vi "02_2.vi"() -> ()   [LabVIEW 2018]
panel:
  out "sum":i16
  in  "String":string="6-7 z: dqzzzjbzz\n13-16 j: jjjvjmjjkjjjjjjj\n5-6 m: mmbmmlvmbmmgmmf\n2-4 k: pkkl\n16-17 k: kkkkkkkkkkkkkkkqf\n10-16 s: mqpscpsszscsssrs\n3-9 n: wlxplcwkkqmdvnb\n16-17 x: mdxqxcxxxtxxxxxxxxv\n4-7 r: hrrrrxr\n3-7 d: ddndddcddddvddd\n7-15 p: rpjvppwfppsppptppqb\n1-2 n: ztznhmhldp\n6-18 x: stxxxxlptpxkxxxxxxx\n15-16 z: zzzzzzzzzzzrzzzz\n4-10 q: qqqpqqqqqqqbkdqrgqq\n14-20 m: mmrmmmmmmfmmmlmmzcmw\n1-2 t: qvxzmfgpxwgkt\n7-11 w: wwwwwwcwwwlwp\n12-13 g: gggsslggggggg\n9-11 v: vvvvgvnvhvvgvv\n1-11 z: tgksdczwmtzsfs\n13-15 t: hrshwjqvtlcqtrtttjhv\n4-13 h: hhhrxhhfhhmhhhhsdh\n2-3 s: shcsssss\n6-14 g: gggwgtgfpgqggwgg\n3-5 t: gsmtttttcbf\n8-9 b: gbbbbbbbbb\n8-9 f: ffqfffflf\n13-14 f: ffffffffffffnf\n13-14 v: vvvvvvvvvvvvhv\n2-8 m: mztxflwwrc\n1-2 d: ddddpfj\n2-7 f: fgffffgfffr\n3-5 t: htjxtstvtspttlxk\n15-16 f: ffffffffffffnfgtf\n3-11 p: pbgllspgppqhp\n1-10 t: mssrtttpzl\n3-4 q: qqcv\n4-5 s: dsscp\n3-6 n: nrjnnk\n2-5 z: zzzzz\n4-6 d: ddddwd\n4-8 f: zfqqdrfwcng\n2-6 s: ssnscs\n4-8 z: fzzzzvgbzwrzqzz\n14-18 z: thmkmmggvkfzbzfzvzt\n2-8 h: hhhhhhhh\n7-9 p: ppppppgpll\n1-2 x: cxkcrk\n1-2 h: lbrhhp\n6-9 k: kkkkkkkknk\n3-4 s: scjs\n2-3 s: fdshfsh\n5-15 s: vssspssssvkrlhk\n6-8 x: xtxxvxzhxxxxtxl\n6-15 c: ncccccccjccfclccv\n3-4 x: xxfcxlxxcxs\n3-8 x: xwxxxtkjxmtlxxxmx\n3-5 j: jjsjljzxjl\n3-12 n: nnlmnnnqgnmgs\n3-6 w: gwvswwww\n9-12 l: hlljlcklrcls\n2-4 x: cxfxqhx\n6-14 m: zrgnffnkcmntszgvnc\n1-6 g: gxqrgnzd\n4-9 z: zpzqzzgzzxxbzs\n10-13 l: jlvlllbxlvllt\n3-4 n: jxnx\n8-10 c: sccccczckc\n10-13 j: jkfgxjjjjjjjjjxzdh\n9-12 h: hhhhhhhhhhhhh\n6-14 p: hvpppxnpkpjbxpppppgp\n4-9 s: ssscsslsc\n3-7 c: cccccgcclqg\n19-20 l: ltfjvlllxhlnnlwlllfw\n7-8 n: nnnnnnnnjnn\n2-5 k: skntkhxkbwj\n3-6 z: pnzzzzz\n5-9 g: gpqtgggwxmghvgrqg\n3-6 k: khkkkkkk\n5-11 l: zlllljllnllllljhb\n6-9 l: lllllllll\n14-15 g: ggggggggggpxgkhg\n4-6 n: lgmntnxshxwpnq\n1-2 s: sxnst\n13-14 z: pwzstpdztzhwxk\n2-3 c: wmqrccn\n13-15 x: xxxxxxxxxxxvqxgxj\n6-8 b: pbbbbbbb\n8-19 f: prbsvkqfcdnrwhlnwfg\n7-8 x: sxlwxqxx\n7-8 p: xdtphpppqpppp\n1-5 p: cgplv\n4-11 k: kqnqkfkfxwk\n9-13 m: qhmnmsmmgmmmlm\n3-5 z: rzzrjxcqpl\n2-7 z: sjzcgsqqtfhnf\n4-7 c: vcpvkbbbd\n10-16 h: dspcrfnrthhvgcmh\n18-20 b: zbbbbbbbbbbbbbbbbbbm\n3-6 b: bbbbbbbbbbb\n2-4 k: kzcmhsv\n5-14 j: djcsjqjppfjwsjb\n16-20 g: gggggggggggggwgggglc\n3-4 g: gqggt\n4-6 l: llfjwr\n7-11 v: vvbmvlvvhbsvx\n1-18 p: nvwrgkkhschlrbbhkjqm\n11-16 z: zzzzzzzzxxfnzzzqzzz\n6-12 f: bxfsflvhfdrgftfsxvf\n5-10 r: trzwrbsrqr\n4-8 g: zfphgnjlgsbc\n16-17 v: vvvvvvvvvvkvvvvkv\n12-13 n: nnnnrvnknvnpdn\n5-9 x: xxjxxxxxw\n1-3 z: szxzz\n3-4 c: cccxc\n12-14 p: ppppppppwppppppppp\n19-20 p: pppppppppppppppppppt\n9-10 n: nnmnnnbnnnrmnn\n6-13 d: dbzdmdddvmdctwdbt\n5-9 j: jjjnjljjngkjjj\n5-8 q: qqqqhqqpp\n6-7 t: tssbttq\n13-14 r: rrrrrrrrrrrrrr\n2-6 w: wxwwmwww\n5-7 w: fwwlwwrw\n7-15 v: vvvvvvqvvvvlvvqvvsvv\n11-15 z: zzzzzzzzvzzsgzzgz\n8-10 f: ffffffffffffff\n9-12 p: pmrppppppppw\n3-5 f: kfwqw\n2-3 q: bkbqw\n9-10 m: mmmmmmmmvm\n5-17 f: wfqfnffffjwfvfffjbf\n9-10 m: mkmmpmmmbkmqmmm\n2-5 h: hhhthhk\n4-13 r: cklprhtqglcrhhrmqsc\n1-3 w: lwqw\n5-7 n: lmxnjknnlnnvbqw\n4-10 z: dlcpzqvjjq\n10-11 r: rrrrrfrrrrr\n2-7 h: hqtmfptxhk\n11-13 g: zmdlpghbsggbglxcjwc\n1-3 c: cnch\n4-7 k: kkknkkkk\n4-5 f: jwtffcfdff\n1-10 j: tjjfjjjzjbjjwr\n11-12 j: jjjjjjjwjjjjjjjjjj\n13-15 x: xxgxxxxxmxxxbxcx\n11-12 d: dcdddtdddddcdddj\n8-10 k: kpkkkkqkmkk\n5-6 h: mdmhjhhrhhdhhh\n13-17 g: ggggfgkngpggrgpgclg\n14-15 b: bbbbbpbbbbbjbsb\n1-7 x: wcqddxxhgmxxxvn\n8-10 l: lllhqlznjlllcll\n6-8 n: rnnnscnq\n14-16 m: fmmbmmmgmmmmmpmm\n5-6 c: vccccc\n7-10 h: vwgnhqhqhgpchhwhhhf\n2-6 n: ndwnnn\n1-2 v: vvvtr\n10-11 l: lllllltlllgt\n12-14 x: xxxvxxxxxxxxxx\n5-7 n: snnnnnnh\n3-5 l: rllmn\n9-12 s: jsssgsssftsvsss\n1-4 r: rfrrf\n6-8 r: rrrrrrrr\n3-9 g: rgpdqgsbfggflgbp\n1-15 t: tsbtrptnrtqtvtlgpt\n8-9 b: bblbbnbsbb\n11-14 g: ggggggggggwggcg\n4-5 c: scwgs\n8-10 d: ddkdxddddq\n2-4 m: gmmm\n3-8 k: wrkjkczkkgc\n3-4 h: sjhh\n2-13 t: tvttttttkttttttxctt\n5-8 p: plzpppppp\n6-7 q: qqqqpqxq\n14-18 r: rrrrrrrrrrrrrrrrrrr\n16-18 w: wwwwwwwwwwwwgwwmwd\n4-10 s: ssssjssshss\n7-8 f: fffhffgcf\n2-11 s: sdszssssqsntsz\n2-5 z: zzjjzw\n10-11 k: kkkkmkkkkzkk\n4-5 l: lllcdll\n1-4 q: qlrt\n7-8 c: cccccscc\n9-10 k: sxgqvkkkkkkkkzkk\n5-9 n: nnlkchnnnnwjn\n6-7 v: vdwvfdcbb\n3-5 q: bmqwtqkdbxzdm\n3-7 h: hhbhhhhhhh\n14-18 q: qqqqqrqqfxqqqqqqqq\n4-12 w: ndnwwcvfthhn\n4-5 b: bgbbn\n9-10 j: tjjjgjjjgjjgj\n3-4 s: svsm\n1-2 q: xfqqt\n7-8 p: fdpjsvps\n4-6 x: xpxxsxljlxxrxqjxp\n4-8 w: mbvdkwwwwwwhghlhj\n1-3 g: fngjxdc\n2-3 j: xtjjj\n4-9 j: lqphjhmgzjzjjvjjtv\n6-9 z: szzxzzqzzz\n5-11 c: cdccncccwfxc\n8-9 t: bttttttvtt\n5-11 l: rttpvrclsqfk\n3-18 b: hlwzvtqbbzbbbbvlvhb\n15-17 f: fffkffffffffffbffff\n2-6 l: lllqlt\n5-9 h: hhhhjchhhh\n3-9 x: xlgxxxxxr\n6-10 n: nnwxmxnpnf\n2-3 l: drlwrtltw\n1-2 b: gxbbrklvbsbbxbbb\n11-13 q: qqlvqqqqqqqqqqqqfp\n1-12 t: thdtvlgbstttmhgttbnt\n2-4 l: lllpvll\n3-16 t: lttpfnrgwdlkqtwgqrj\n7-8 d: ddddtdddd\n10-12 w: wwwbwwjwnwqwbwswwwg\n2-4 c: qqct\n1-4 j: jcjrjj\n4-5 l: lllbll\n11-16 g: ggkrgswgljjggmpzkg\n7-11 b: rbrbbczsbbbbbbfvck\n16-17 r: xfnpkmnzmlnrwrrrr\n8-9 x: xxxxxxxjz\n6-10 p: dpppdptpbpxpgbpppn\n4-5 s: scvcjsqssbs\n3-4 k: kktv\n8-10 f: fffffffffs\n3-4 g: gpbq\n10-11 x: xxxxxxzxhgdqxxvxxxxx\n7-8 g: nzgpgxgv\n4-6 n: nnnbzsnbh\n3-14 l: jdllllltlfjlld\n7-9 v: vvvvvfvvv\n5-7 s: ssbsssxjv\n6-11 l: xlllslrnlflnqhklllll\n14-18 x: xxxpxxxxxxxkxxxxxx\n10-12 x: xxvqxxxfxjxxxxxqp\n4-6 h: xfhhhhhhhj\n2-3 b: rbbbjmb\n7-10 d: dddddddddd\n15-19 g: ggggfgggjgggggggghg\n1-4 t: stth\n7-10 r: zskrphxkhgtmnsmzlr\n9-15 d: tkbdgngsddddrcd\n3-10 q: krqsqljqdfzqqq\n4-5 t: tztxtrgt\n11-14 z: jzzzzzzzzzzxzz\n18-20 p: pxpppbpppppppppppppv\n10-17 t: tttttjtttdtvvfqttxft\n8-15 j: vbjcjtdjzsjjjwjj\n4-7 d: ddddddd\n5-6 h: vmhlhj\n9-12 h: rhhrbhhhhhjh\n3-5 k: lkbkk\n6-11 d: dkfsjdmdddn\n7-11 d: dddddrsdddqw\n2-4 n: wnxngd\n12-16 c: cccccccbccccccctcc\n7-13 f: blfjmffffffwlf\n14-16 s: zsssssssrssssslrzfps\n5-6 t: tkkttt\n7-13 j: xjkjjrjmxjfpnvxqj\n8-14 c: cccccccckccccccsc\n11-14 k: kkknkkkkkhkfkxnkck\n4-5 d: ddddd\n4-5 w: wzmwwwww\n12-13 r: rnrrrsrvrrsrrrrrrr\n6-18 p: ppjppppppxppppppjppp\n1-5 m: gzhfjm\n2-5 s: scsrsssv\n7-10 t: tttthmztxbt\n3-8 c: crccmpwc\n9-11 f: ffffwmvffzfrzkfff\n9-10 q: vqvjtbtqkcnsbmfl\n4-10 l: lltlnfzxglwfxpgwntj\n2-3 c: pcccc\n5-11 s: jjgxwdfnsgjgxk\n3-8 d: vjqsdvjdhsx\n1-11 t: bjpthttlzttpbxtds\n7-8 s: sssssxsss\n2-6 b: qbzglpffcldtdb\n5-7 c: cccccvc\n5-6 f: fvffffz\n6-7 s: sspssdzhswsn\n1-6 l: wgdppqwnqp\n14-15 b: bbbbbbbbxbbbbbbb\n2-11 w: vqwtkmvbgrp\n5-7 w: wtwwwwwwwwww\n4-5 s: rsssss\n1-4 t: bwttt\n9-12 m: mmmmmfmmmwmn\n3-10 s: gmgjdslsnwsrv\n1-4 c: zsfcsrvsxczrgbtpwjkv\n11-12 f: fgffgtrfffksfff\n6-8 g: gggglbgg\n7-10 c: crcjtcccbh\n6-8 t: vjdktttttzcnthtwvtvb\n7-8 h: hchhthqhh\n4-10 k: hhkknpdlfk\n3-4 r: rrsjr\n7-11 g: ttrjggkdwbdnzmwzd\n5-8 b: nvqpcvfb\n6-9 b: bnbbbftbmbq\n1-4 m: smmmmmmmmmmmm\n16-17 p: pppppppppppphpppp\n10-13 f: ffwffffvmthvp\n9-12 n: nnvvcvmmfnnqnnsnnnn\n2-4 r: rrwq\n2-9 x: xzxxhxkxxtzdc\n6-7 t: ttrtltxt\n4-5 f: fffgxf\n3-6 v: vvvvvm\n5-11 m: mgxzmmgmlxxmm\n3-4 n: knnjcxn\n3-4 d: dndkgvkpbhdddcpt\n6-7 x: nxxxxtd\n11-12 k: kkkkkkkkkkmkk\n7-8 b: bkbbbbbzbbfmj\n2-5 d: drtdq\n8-9 q: qqqqqqqzj\n7-9 m: mkmmmmzmpfm\n3-5 b: bwcbv\n2-4 v: vvvvvvv\n5-6 h: hhhbbv\n12-15 g: gggggggdgtgqggngg\n8-9 l: llldllllll\n3-11 f: fdfpflzwfffct\n5-6 z: bhbzjgzz\n5-18 r: jtmnrhfrsptklgdksr\n7-9 d: llcrcqsfc\n16-17 l: kllllbllllllllllll\n9-15 g: ggvtgvgjggmgwslggm\n4-10 g: ggggggqgggqggp\n3-5 c: gchcc\n6-11 z: zzzzjzzzzpz\n3-16 h: hzhhhhhhhhhhhhhhh\n3-8 w: wwqwwwwdw\n3-4 g: wmklgdxxb\n2-5 p: ppbwqsg\n1-3 p: xpvpppppp\n13-16 x: pfqxdnxwxxzpxxvx\n3-8 m: qmlhjkzhm\n8-10 l: llllllfllll\n12-16 p: xtppfpfppppppdlk\n7-10 t: ttttttztmt\n11-13 p: pwlphpppcwnpv\n1-3 x: xxxx\n12-14 c: hcckccccccbvdz\n3-8 g: ggggggngg\n11-13 b: bbbgbcbbblxbbbbbb\n2-6 k: kkhhlhvtbd\n3-4 s: sstsss\n13-16 l: nljgklqlgfrlljtl\n9-14 l: llllllgllllhln\n3-15 b: bbtbbbbbbbbbbbpbbbb\n7-10 h: hhhhhghhhjh\n4-6 r: pnxrvrrnwrcrrw\n17-20 h: xbhcmhpvqzlhrbhhhbjn\n1-4 f: fffff\n2-4 c: vcclc\n11-14 f: fffgnffflffffff\n8-15 s: ssslsscwcssszsv\n7-10 r: drrbvtrphzqqrrsvncr\n12-13 l: vllllllllllbfl\n7-11 z: zwhzzhmqnbj\n6-11 v: vvkvvqhvvvjvwvvvvvvv\n13-14 h: shshhmhhhhhhfhvsr\n5-10 c: rwzcxwzvgcpn\n4-7 f: ckdfpmffpzlwjl\n5-7 x: xxxxkxgxxx\n18-19 x: xxxxxxxxxxxxxxxxxkxx\n4-6 r: nrcrdgrbrb\n9-12 f: ffffffwflffff\n5-10 z: zzzzzzzzzwzzzz\n4-5 d: dqmvqlhjxdkkdfn\n10-15 s: ssssssssssssssssd\n8-10 w: wpjvmwqwwz\n6-10 w: hxwxcwrqbb\n9-15 f: fffffffffffffbftb\n5-7 q: qqqqqqx\n3-5 t: wgbttttp\n12-13 k: kckkkkkkkkksztk\n12-15 w: wgwwwwwwbwwwwww\n2-3 s: tssstcph\n4-7 l: llllkll\n6-7 w: wkwkrxsj\n3-4 w: wkwwfm\n3-10 w: swtwckrrkwrvk\n5-6 w: wwwwwwlwjkknh\n1-3 d: dddd\n1-2 b: bcbj\n8-10 f: fffffffbvbf\n7-12 d: ddgvftsdrffbtd\n5-9 f: fffffffffffftf\n4-11 j: rbhjbkfjznjwqwz\n3-9 z: czzgzbhvz\n9-12 x: xxxpxxxwjxxvx\n3-9 k: zzkfjkcfk\n7-9 f: tffqcfgfvlffmd\n2-4 j: njzn\n9-10 h: hhhhjvhhhhh\n3-7 n: hndnbjdjx\n1-2 s: sshfsss\n7-14 g: kglngzbggggnvcgtgt\n11-13 h: hhhdnfhhhhqhhhhh\n5-6 w: twwwww\n5-8 j: fgxbqjjh\n7-8 f: fffffhvp\n3-9 j: pjjjjjpbj\n3-4 m: vmmsm\n12-13 x: xxxxxxgxqxxjnnx\n4-5 t: ttbbtt\n10-12 p: jjpppppcppppblpp\n9-10 b: wlbbbbjbbkbgnbbb\n6-8 t: tttstttzt\n6-9 n: fqxlnnnmn\n4-5 k: gwdzkk\n4-11 t: ttthktthtttbt\n2-4 r: rrpcnhrktrl\n7-9 j: hjbxdqbbmxmm\n3-7 b: bbbzqbbsbh\n15-17 s: sssdssspssssssgssss\n6-11 w: wwwwwpwwwwdww\n14-16 s: sssssssssssssgsrs\n2-8 z: kzbzbzthzgzzwcw\n11-13 q: qqqqqqqqqqjwq\n3-4 v: dspkvr\n1-5 n: nnnnnnmn\n4-5 b: blbbsbb\n5-7 r: rrfrkcr\n5-6 c: zpcrlp\n15-16 b: bbbbbbbbbbrbbbbg\n5-6 j: jjjjrcjj\n9-12 z: mzgnzzdjzzzzzdzlzzzz\n5-7 z: gztczpzbzdzlzcjzj\n6-8 w: hwhwfmswrrcpxlsqlkkd\n6-11 p: pppsppmpnpp\n1-2 w: vdwl\n8-13 m: mmkgmmlmnmmvm\n2-3 q: qqqh\n2-5 x: xxxxrmxxxxxjxnxxcnd\n7-8 p: fwpppptp\n2-10 l: lllbhlltclln\n10-11 v: vvvvvvvvtrgvv\n13-16 m: mmmmmmmmmmmmnmmmm\n3-4 n: qtfn\n7-8 g: gggwgggw\n10-12 n: xnnnhcqhnnnpnphnnnnx\n3-4 q: qrqq\n4-8 c: cswcccclzx\n2-8 h: hphhhhhd\n1-16 r: qrfrfrtgrrrxrrzhbg\n11-12 q: qqqqqqqqqqqqqqqq\n10-11 v: vvvvvvvvvdf\n6-8 n: lnnrnnwnnldmwn\n1-5 j: jjdkfgkjvjjjjj\n14-15 j: jjklzggckqksgvk\n10-11 g: ggggggggnzng\n15-17 n: ntnnllvnmbzwnnhzw\n13-16 g: gggggggggggqdgghc\n12-16 g: sgggggggglggnggggggg\n3-4 x: xnplx\n5-9 m: mjldmlmmmgbmjsbkm\n18-19 h: hhhhhhhhpzhhhhhhhhh\n9-10 f: ffbfffdfjf\n8-13 s: gssghjssgxsgssgsnj\n2-5 m: mmmmbhdzkmmh\n8-18 l: hqnqzznqkmskljggbl\n2-3 m: nfjm\n1-7 z: dnztzkpfwv\n2-9 s: ssvsdvjwdsw\n15-19 f: fffffffffffffcsffcn\n13-20 c: ccccccccccgccccwcccc\n3-15 b: bwmzdgbbjvbbbrt\n10-13 d: ddddddgcddmdhdd\n4-7 h: hlhhhphz\n2-3 c: cccbgfbzdql\n13-14 w: wwwcwwgwwwwwcqwzw\n2-4 m: hmmlmmmmmm\n3-16 x: jzxcfkxzxcvfxwxfxx\n3-8 f: kfpffvfwfkf\n8-10 q: pqqmlqqcqqqqf\n3-6 r: qrfcrrwqcrrbttrb\n3-10 s: kdstdvqqdcb\n11-12 f: lcxfllffffffflffff\n4-8 m: mmmmmmmzmmmmm\n6-8 w: wwwwwswwdw\n10-15 b: bhfbbjclbbhwthxltsjn\n1-5 v: dvxvw\n13-16 s: ssssssssssssksswss\n6-7 d: dlfldrt\n4-10 x: xxxxpxqxgxgrh\n4-8 x: xxxxxxxxxx\n4-5 r: vrxrrrrrkxrp\n3-14 h: hfmpnxlklhhhjhzh\n11-15 d: cgddqnxgddddzrdd\n7-12 v: csmfvjvlvzjv\n4-5 g: ggngh\n14-17 z: vzzzzzzzzzzznvzzzb\n15-20 q: qqqqqqqqqqqqqqqqqqqn\n1-3 x: xbxqnzhjzhbxbbnsnt\n11-13 d: sfdtlhdddjkshd\n11-13 c: vbtcncclfzmcc\n1-7 t: ptttttqtt\n3-4 x: xxsxx\n1-2 h: hjhh\n10-13 f: vlcfqpwgqfthf\n14-19 w: wtswwwwwcwwpwswwwww\n7-10 h: fhxhhhhlbw\n4-14 k: khfkkckvkdxkfkvp\n4-6 k: kknkkkbk\n3-14 m: mhvdmpnmwvkcmgbbv\n17-18 h: hhhhhhhhhhhhhhhhrs\n16-18 c: cclccccccccccccxcmcc\n9-12 j: vjjjljjjqjjjjq\n2-3 d: dlrbddmj\n10-15 l: lllmlllhllllllll\n1-2 n: nbnd\n8-11 b: wvbbbbdbbbbbpxbbb\n4-5 c: mccccfcc\n2-12 d: kbdsddgddpwddzx\n9-10 t: ttttjttttbtt\n6-7 j: jjthjvwj\n2-7 l: lglqllxlh\n2-4 t: tnqjb\n1-8 c: nqrbcgbchxwkjrxv\n13-18 c: ccxmccccccccdcgccn\n9-10 s: shsssgsgssksl\n4-9 n: nnnxnnzngrpxn\n10-14 x: jprjxdlnrfwnqx\n1-5 b: bsshbls\n1-4 n: nttnmbblbntbssqn\n8-9 x: xxxxxxxxxxx\n2-4 c: nnccmp\n1-14 t: stttztttttlttq\n9-16 b: rfbmptrnbhwbrgbbqb\n1-4 f: rzzfjkmnwlbnrqmfns\n1-3 x: mxxdlxnklrktlgzd\n3-13 v: zlnktcwvmkqsvjvnwzv\n1-3 r: rrrrr\n5-7 d: qdddcddldd\n2-5 t: tnttktt\n8-15 n: ngnnnnngnnnnnnn\n1-2 v: vfvn\n3-17 f: ffffjfffffffffffgff\n5-12 x: nxxxxxtxxrxxx\n2-14 g: nfgvdgnhggrgtkv\n11-12 k: kkkkktkskkkkksm\n15-16 c: rccccccccccccccccc\n10-12 l: cllwldllplsl\n15-19 b: qbjbpbbbbbbwbbgbbcq\n13-16 f: dqcfgwfffffffffb\n3-4 q: qtzj\n13-15 z: zzzzzzzzzzzvzzzz\n13-18 q: qqqqqqqqpqqqqhqjvqsq\n7-12 r: dtflckrndscrqrcclxb\n4-9 s: zqsssshqscs\n2-5 s: ssrhsfsszsc\n7-8 k: kkkhkkwzktkkk\n17-18 x: xxxxxxrxxxxxqwhklp\n16-17 k: kkkkkkkkkkkkkkkkrkk\n9-11 s: szqfssvgfvm\n11-17 m: mmmmmmmtmmmmmmhmpmmk\n6-7 l: kgllhjdllwqvllnlcn\n1-2 g: gghgfgv\n4-5 f: qfrrrlfrtfzgfct\n6-7 z: zvzzzzj\n7-12 m: lmhzrxztktzpkvw\n3-4 p: ppxpp\n4-5 c: wvxch\n9-12 x: xcxxxxzxcxpxx\n10-11 t: tttttgttttl\n2-3 w: tcwdwb\n1-8 m: mnsmmmmgmm\n1-5 z: zzzzz\n2-13 j: jvjjjljjjhjjjrjlj\n4-5 s: kcmxszckjcsswjbsxn\n6-7 j: dhjccbb\n15-19 x: xxxvxnxxxxxxxxnxxxx\n15-18 f: ffffrffsfffffjffsff\n8-20 m: xmcwmmmhsmmmmmbmmmmm\n8-14 m: mmmmmmkmmmmmmm\n2-6 r: bnrrrv\n8-12 k: kkkkkkkjkkkpkkkk\n1-4 f: flqfgnffzjrfz\n2-6 p: pcvgxpnl\n9-12 n: nnnnnnnnkgntnn\n13-15 h: hhhhvhhhhhhthhhhwphh\n6-7 h: hhhhhhkh\n8-9 h: vhhhhhhhhh\n1-5 m: mbmmmszqwmxdhd\n5-6 v: vvmbwvv\n4-6 g: vggttg\n8-15 t: dzkznmcvqmbbtxs\n13-15 j: jjjjjjjjjjjjjjjj\n5-11 r: ptwmxlrttvxk\n10-12 s: ksszsbqxsjsssnjst\n3-4 k: jwkr\n3-6 m: mmtkmmm\n2-4 l: lhlll\n7-12 p: pppppprppppzpp\n1-2 n: bznpdd\n11-13 t: ttttttttztdct\n6-12 c: cccccdccccccc\n2-7 n: nznnknrnnn\n14-15 h: zqxhdhhxhhhhhzpr\n6-7 x: xxxxxjx\n5-7 s: gsfcshsbxnc\n12-13 j: jjjjjjjrjjjjjjjjj\n4-5 v: vvvvc\n4-10 r: rrsrzrhrrgrmvrs\n8-12 c: cccwcccccccmc\n4-5 v: vvvvv\n13-19 j: lfnkrsjjjjjrjjzgcmj\n3-4 k: kkskkk\n11-14 s: sssssssssssssssssss\n8-9 k: kkbkknkkk\n4-6 z: zzzqzqxzz\n2-4 f: rgtz\n4-13 k: kkkkjkkkkkkxk\n1-6 q: jqqqqpqqqqqqqqqqqq\n7-9 b: bbbbbrlbj\n4-5 j: mgjjtjfs\n15-16 p: ppppphppppppppnpp\n2-3 b: btbt\n11-12 v: vvvvvvvvvvzk\n1-4 b: qbbbh\n6-7 b: bsbbbbnwb\n3-10 j: gkjrhtjjfjjjrjjjjrw\n4-5 g: gdgqtpgg\n15-17 g: gggggggggrgggggggg\n1-3 j: hjdjpj\n5-6 k: jjslkhnwkfqjprk\n7-10 s: ssscssssnsx\n1-9 n: nnnnnnnnnn\n1-14 t: ptttttttttttttt\n11-13 q: qqqtqqcfvqsxzqqqqqq\n14-15 r: rrprsrrrqmjbrrv\n4-5 h: hhhhdhh\n5-8 l: lllllllll\n18-19 f: fwfffffffffffffffff\n9-11 j: zjnjjvjjfbj\n3-7 p: sjpsmsc\n10-11 s: sscsssssrrls\n3-9 q: qqqqqqqql\n6-20 s: sqscdsmdgvddfsvprgcs\n18-19 q: qqqqqqqqqqqqqqqqqqq\n4-5 g: mgjggnjfgl\n3-5 p: ppcpzp\n14-16 t: fjxbttlttfprttlt\n4-7 v: pzmvzvlzxcccvmvvwfdb\n1-8 r: rkrrtkrrgrrq\n1-10 h: qhhhhhhhhdf\n1-4 p: rpppp\n4-6 s: skshzg\n16-17 h: hhhbhhhhhhhhhhhch\n2-10 m: mrmpvlsxvtlkwpnl\n7-10 b: bbbbbbbrdb\n15-18 j: mjjjkgmjjbjjjjcjjmjj\n3-6 m: mgmmdmmmj\n5-11 n: ktnnwnnntznqnnnpnnn\n9-12 w: wwwwglwwzwwtww\n8-9 t: ltttvttvv\n4-8 c: xdfklzfhgjgcktssk\n7-11 x: xxgxxxxzxmxxxxqcc\n13-17 v: vvvvvvzvvvnvvhvbtv\n13-16 c: ccccccccgccccccw\n3-13 m: mmkpmqjkdknmmrmfcm\n7-11 g: gpgsvmgvdkg\n9-14 g: gvgglglghgjpwjzgsfh\n2-3 v: vvcv\n3-8 w: zwqjwwwwwm\n7-9 k: kkkkkkzkb\n3-4 v: gvvk\n14-15 r: rrrkfhmpgbhtqrh\n4-5 n: nnnmwnn\n7-9 l: llltdlvlx\n6-7 f: ffffffl\n7-8 n: nmnnnwfg\n17-18 x: xxxnxxbwxxbxxxggvxx\n1-3 z: cbzntpzvgpszsdq\n3-4 j: jjjj\n3-5 z: zznzgz\n4-5 j: jjjcg\n7-8 j: mjjkjjxhj\n1-2 t: vrlmttt\n3-4 h: hhhhhrhhhphhh\n14-20 q: qqlsqqqmqqqqqqqsqjjg\n9-10 r: rxrrrrcxrbrrnsc\n8-15 x: ghlzxrvjvjxrndvknxxt\n1-3 b: bbbb\n4-6 t: fnqthtnfjprghdmt\n6-7 m: mmmmmcgmm\n6-8 q: bqqvqvqd\n7-16 v: vvvvvvvvvvvvvvvvvv\n3-4 p: ppjlppppppppxlztpp\n12-14 g: ggggnrggvgggmgg\n1-10 k: kxkktkkkpkkgt\n4-5 z: zzwrw\n14-20 p: pppppppppppppspppppp\n6-11 t: hkbbtbmrdlkjlthgkc\n6-13 f: fpcfzfcpfjqhqwffffd\n2-3 h: hhhjhh\n3-4 z: ztcbz\n6-9 q: kqlqgtqwvxcgqwqr\n9-14 k: kkkkskkknkkckjk\n14-16 n: nnnnnnnnrnnncprcnn\n1-9 m: pwwmgmxmnmm\n1-5 f: fnmpfc\n3-5 s: jmsls\n5-7 b: bbbbbbbbbbbj\n4-12 m: gjzqmjktbrbk\n4-5 k: krkkkk\n3-10 q: qqcnrqqqbnqq\n1-2 s: gvsk\n5-6 n: nsjnnn\n1-5 w: wwkwztqc\n4-17 z: zbbnqfqmrjbszpwxz\n2-9 z: djpdvrdbx\n2-4 w: lwxw\n1-10 g: gsgpgggrgggtgwsgg\n3-6 q: qqtqqq\n3-7 x: xdxxxxx\n1-2 t: ttft\n4-6 x: lxjxsxpvxxxkjqlsxndf\n1-8 r: rbzrrrrrrsrrrrrv\n1-6 g: gggggggggggggg\n2-3 q: smbbmntqr\n8-9 d: bzmplgdfq\n5-10 w: wwwdwzjwwwww\n2-11 z: jzgphzdjwxw\n9-12 d: dtvdddjdlddddd\n5-16 s: hswkqwssjshpsxkgmsw\n3-13 c: cwbcccccccccgc\n2-13 b: bhswhcxchtknt\n1-3 h: hhhtmclgrtxdvqfpk\n12-13 w: bswxxxmxwjtwp\n4-6 c: xtcccc\n6-16 k: msskfkgdkpcnqtzkpqh\n6-7 t: tpttftt\n5-7 h: hhhhhhh\n3-8 t: tbrshhlt\n8-10 j: jjjjjjjhjjjjjjjjj\n11-13 g: vgwggggggkshjggnqggs\n6-10 q: jqqgzqpwqqfqqqd\n5-12 d: ndwgszjhhdwv\n4-5 t: tttmkttt\n2-3 p: ppwp\n7-8 t: ttttttzb\n13-14 m: mmmmmmmmmmmmpxmm\n5-9 v: cqvbqvzzvtcdnvvvbz\n10-12 q: xbfpjqpzlqcq\n8-10 l: lhlkllclll\n4-15 t: wjtqftxkskpvttxmb\n1-5 s: lzscqfrpfss\n7-9 x: xmvxfxxjx\n6-7 w: wwwmwwwwww\n13-16 d: kbddtmrdqgqqddhd\n1-17 q: vqqqqgqqqqqqqqqqqqq\n3-5 f: nkftsfvzc\n4-7 h: hhhhhjrd\n5-11 z: zzzzzzzzzzlz\n4-7 k: kkkkdkkk\n17-19 n: nnnnnnnnnnnnnnnnwncn\n8-16 r: hpvsmthdvmxrbqvr\n2-10 b: bbrxblvbbdvcbdbbbqsb\n8-11 r: rrrrrrrzrrv\n1-2 r: vtrr\n2-3 m: mmcmmmm\n3-10 c: xccccscccc\n10-11 w: wwwwwwwwwwzw\n3-18 f: fspffffffjpfffffff\n4-16 q: kqqqqqqqqqqqqqqkqq\n10-11 l: llllxlllldv\n13-19 t: ttttttttttttttttttt\n9-12 d: drddddddmddd\n5-6 n: kngrnn\n5-9 x: sbxxxtkvpjfxxxv\n8-11 d: dkwddrdrdddd\n8-11 d: ddsddddhdbd\n4-5 l: pxlll\n12-15 m: sjlnmmhndcmmzrmm\n7-9 t: ttttttdtctt\n3-5 n: snfxc\n4-5 l: lmpll\n5-10 z: zzlztzfttxzfprz\n13-14 d: ddwjdqvjdddvdj\n14-18 r: rrrrrrrrrrrrrgrrrhrr\n4-6 g: ggggqc\n9-16 m: mmrmmmmmmmmmrmmm\n1-8 f: fffffpfkffff\n7-8 b: bbbbbbdtbbb\n5-8 k: hkkbkkkkkkwk\n9-12 d: dhdddqdhddkddddddd\n10-12 r: rrcrrxrrrgrr\n6-7 r: rrrrrrrrr\n12-18 c: cccccccccccccccccc\n1-3 x: glnwxx\n4-12 s: splscqfbvbvswgrvvhg\n7-14 n: nnnnnnpnnnnnnb\n4-8 x: xlqxbrkx\n11-13 t: ttttttttttktv\n1-7 w: wwgwwww\n8-13 p: lpzxtppplplff\n6-7 q: qqwpkqqqqz\n4-5 j: zdkmjrpjlzbjprv\n4-6 x: xhtxxxg\n2-14 j: jjjjjjjjxvjjtjjjwj\n8-9 d: gddddndcgtdn\n4-7 g: gglgpgr\n7-10 d: drddddsddd\n1-3 n: nbnnb\n3-4 k: dggss\n6-10 t: cwcwtnttmt\n3-4 x: xxxx\n8-12 t: jttmtbttqtztttzmtc\n8-10 t: tttgtttztttg\n3-4 h: hhhhc\n10-18 t: tttttttttmtttttttbtt\n3-5 n: nnnnnnz\n4-12 w: wwwwqwwwjwwxwlwqww\n2-4 x: xqdpr\n9-16 k: kkkkfzbkkkknjknkkr\n2-7 t: tttttwt\n2-4 p: npjp\n5-12 c: cccccccccchxcc\n9-14 x: xvbxpxxshxnmxzxxxwn\n10-11 t: ttqtvttjtcttmtttt\n9-15 c: cccbcxcswnrzchfcqwjc\n3-4 s: vpczjdzgfsqnpsscf\n7-11 b: bbbbbbtbbbb\n4-15 q: qqqzqqqqqqqqqqqqqqqq\n2-4 s: fsvsmlsfbgz\n1-8 w: wbwwwwwtww\n8-9 w: phbxcfdwwhrbhkgrzdx\n6-9 x: xxdpxhsxxxkx\n5-9 b: bbbbfbbbsb\n12-18 m: mmmhmbmmmfmrmmmmmmmm\n12-14 l: lllllllllllllll\n8-11 z: zzzzzzzzzzzzzzzz\n2-3 d: dlld\n6-7 b: kghbbbbbg\n18-19 c: cccccccccccccrcccccc\n6-8 m: mwnpmmjmfmmmfmhjf\n1-5 j: gjjjxl\n3-4 p: pzpppppp\n12-17 z: zkzzzpzzzzzndzzzzzz\n13-18 k: knvkkkzvkkkkkkwkkmkc\n3-4 h: hfgrm\n2-6 z: xzzzvzkzzzzvprtgz\n12-19 b: bbbbbbbbbbbpbbbbbbdb\n3-11 v: xvrvmvvvfgzvjv\n7-10 r: frrrcrrrrrrzr\n1-17 v: vhpxjwbpkcctdpsvfkxs\n3-8 d: hbdzlkdk\n5-6 f: flffzf\n2-4 s: ssnsssh\n4-5 m: qmffj\n6-11 z: zzzqztznfzzkc\n3-4 m: tjkm\n2-4 n: nnwn\n4-5 s: npxck\n16-17 n: nnnnnnnnnnnnnnnpk\n10-12 s: ssssssssssss\n2-4 g: twghtgs\n9-11 w: wwwwwwwwdww\n15-18 h: gfvmkzsrczchxwfvdr\n9-10 p: ppppppprtp\n4-5 p: pppgf\n2-11 c: qccccrsbjbsxbnjx\n8-9 l: lllllllvl\n10-15 s: sksssssssssscssss\n4-8 k: kfkklhgk\n5-9 t: ttgndtthqcfj\n2-3 t: spntttnqdttjt\n12-16 t: tttttttttttttttttt\n19-20 j: jnjdjbzjpjjnjjrjjjdj\n2-6 c: rrbhhggnnzcjvp\n7-13 r: rrlrrdrrrrrrr\n2-8 f: dfsvpmqfbqc\n10-12 p: bpprppnbprpppp\n4-6 z: lzszznzzxxzzm\n2-5 v: vmvvv\n9-17 v: vvvvvxvvvvvvfvvvf\n6-10 t: tcflkttctht\n10-16 d: qbxwwbqdxxlqtndktlx\n1-8 g: ggtgggcgggggr\n1-2 t: tttqqt\n9-10 k: knkkcnkdkkzkkkq\n12-18 r: rrrrrrrmrrrrprrrrkrr\n2-5 x: xxxcxxxxxdsjx\n6-7 z: cvzzzzz\n5-8 b: qjpzdbdx\n19-20 n: nnngnnnhnnnnnnpnnnwp\n3-19 g: vgggpxgnfkhvdrgggsng\n3-5 b: bvbbqh\n3-8 h: hhghhhhhhhhhhhhh\n2-4 x: xxtxfcppsvxrdtnjgs\n6-8 x: xxxxxxxx\n1-4 k: kfzkbkkkt\n17-20 h: hhhhhhhhhhhmhhhhphlh\n5-7 b: tfbvbrc\n2-4 f: ffcgfzfrmfsft\n18-19 t: ttfttqklqvgtkltnlgn\n1-4 c: tctc\n8-18 g: gkndqqgdgqrgkzgggg\n11-12 b: bbbbbbbbbbbpb\n5-9 t: qgtntdbdw\n1-5 n: nqnnnnkns\n1-3 c: bcccqccccw\n8-13 l: lllllmpkllllwhl\n7-10 c: czcsbcnccqwcsgxpcw\n3-5 h: bhhqjjpnh\n9-10 p: pppppppppw\n4-5 x: xxxxf\n1-5 h: mhhhhhh\n1-17 c: hcccckccpccccfccc\n8-9 p: pdgpplpppp\n1-7 r: rrfrrrmrrr\n3-18 x: xxxxxtxxxxxxxmxxmlx\n1-4 t: fttt\n9-14 x: fxxcxmzqgzzjktddmcf\n3-4 t: tttt\n3-5 l: lljmk\n1-3 g: dswcw\n7-8 l: ltlxlnllll\n2-4 q: lqvqpjcqfk\n2-7 r: prrrjbrrlmrbb\n4-7 b: bbbbbbbb\n5-6 k: krhkkkkkkk\n2-6 x: xxxxxxx\n6-12 t: xmttzbtspxgd\n1-8 x: xxxkxhxxxxx\n7-12 r: rrrrrrzrrrrq\n17-18 k: kkkkkkkkkkkkkkkkvsk\n12-15 j: zjbctccpfljrzbd\n9-10 z: zzzzzzzzzmzz\n1-4 l: crmn\n6-15 k: nkknzkkrgkcnkds\n3-9 z: zzzzzzzzzz\n2-10 v: vvvtpkxkvvvvzvvvvvvv\n1-2 h: hhhsn\n2-4 p: qgpgp\n2-4 p: dvqjxdwnvrkpg\n15-16 p: nkprmxpxpxhvpcmw\n16-18 b: qbbbbbfbbbbbbbbnbd\n4-5 t: thtxt\n2-7 g: rpvlhbdw\n6-7 k: kkpxdkg\n7-9 n: nnnnnnqnz\n17-18 h: xnmkfwtzflhkpsjthhbl\n3-5 k: kkdkm\n14-15 h: hhhhhhhhhhphhhchzzt\n6-13 j: jjjjjjhjjjjjjjk\n2-4 x: xxxwxx\n1-2 s: ssws\n4-5 m: fmztq\n5-6 p: ppppld\n3-7 w: wwwwwwww\n5-7 d: vgfddxdzvkndndzm\n1-10 n: nnnnnnnnnnnnnn\n1-9 q: gwmrrblpmqlqpqgqqmqj\n2-12 s: mqspzltmqsngwmlmk\n3-9 w: twhfxnkmw\n12-13 c: cczcccccccccl\n2-4 d: dpdtdqlssxddddddhd\n1-2 w: jqvw\n6-14 n: nnnnnjnnnnnnnnn\n6-7 b: bbbbbbbb\n14-16 z: zbvzzzzzzzzzzzzzzzzx\n7-12 f: fffnfffdfqfffg\n1-2 t: ftttt\n5-18 d: dtcdddjvdxddsdtdkk\n15-18 s: szsssssdsssdhstssp\n6-9 m: lmmmmmmmgljm\n2-6 n: nvsnjg\n5-6 l: lllhvx\n16-18 r: rrrrrrrrrrrrrrrhrr\n1-2 b: qbkbb\n10-18 x: gfjmjtbxxlxmxzxxql\n2-5 c: cdbjm\n3-4 k: rsvvwknnkjvwnkkf\n1-3 b: mbbbbb\n3-4 c: ccccc\n3-4 x: zxtkxn\n2-10 d: dbdddqtdxvjq\n8-11 k: kzkkpkkbkzq\n4-7 h: hhxhzmwhhhh\n11-16 r: rrrrrrrrrrrrrrrlr"
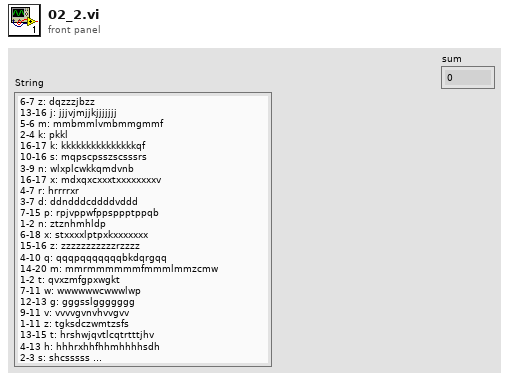
[diagram p1: front panel]
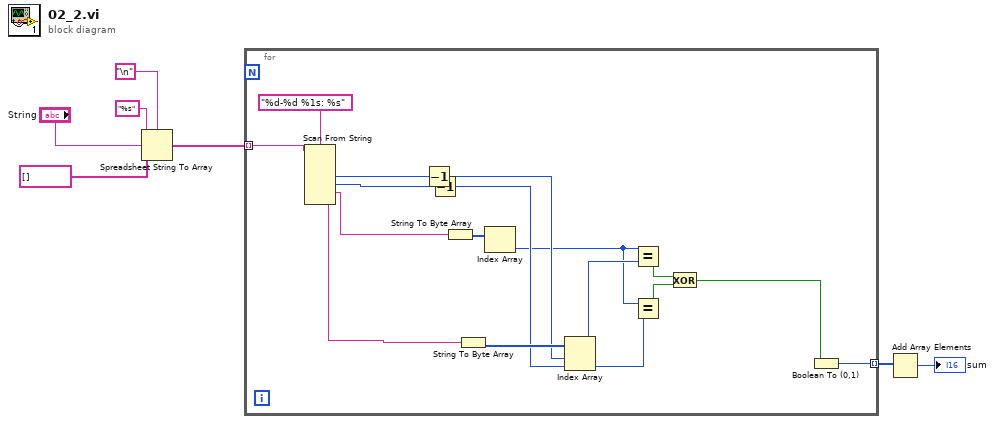
[diagram p0: block diagram]
diagram:
  n1 = Spreadsheet String To Array(delimiter (Tab)="\n", format string="%s", spreadsheet string="String", array type (2D Dbl)=string[] []) -> (array=w3:string[])
  n2 = for {
    tunnel: w3 -> [w24] mode=indexing
    tunnel: [w19] -> w2 mode=indexing
    n3 = Scan From String(format string="%d-%d %1s: %s", input string=w24) -> (output 1=w17:i32, output 2=w16:i32, output 3=w21:string, output 4=w22:string)  [unwired: 6 in, 3 out]
    n4 = Decrement(x=w17) -> (x-1=w15:i32)
    n5 = Decrement(x=w16) -> (x-1=w14:i32)
    n6 = String To Byte Array(string=w21) -> (unsigned byte array=w20:u8[])
    n7 = String To Byte Array(string=w22) -> (unsigned byte array=w18:u8[])
    n8 = Index Array(array=w20) -> (element=w12:u8)  [unwired: 1 in]
    n9 = Index Array(array=w18, index #1=w15, index #2=w14) -> (element #1=w13:u8, element #2=w11:u8)
    n10 = Equal?(x=w12, y=w13) -> (x = y?=w10:bool)
    n11 = Equal?(x=w12, y=w11) -> (x = y?=w9:bool)
    n12 = Exclusive Or(1:w9, 2:w10) -> (0:w8:bool)
    n13 = Boolean To (0,1)(Boolean=w8) -> (0, 1=w19:i16)
  }
  n14 = Add Array Elements(numeric array=w2) -> (sum=→"sum":i16)
